vi "AdamsEncoderTest.vi"(10 "FW2DevRef":T1={"DevStatus"={"status"=FALSE, "code"=0, "source"=""}, "EncoderIndex"=enum."Invalid", "CounterIndex"=enum."Ctr 1", "DistancePerCount"=2.0, "Decoding Type"=enum."4x"}, 11 "FW1DevRef":T1={"DevStatus"={"status"=FALSE, "code"=0, "source"=""}, "EncoderIndex"=enum."Invalid", "CounterIndex"=enum."Ctr 1", "DistancePerCount"=2.0, "Decoding Type"=enum."4x"}) -> (2 "FW2Change":dbl, 3 "FW1Change":dbl)   [LabVIEW 2014]
uses:
  <vilib>/Rock Robotics/WPI/Encoder/WPI_EncoderDevRef.ctl
  <vilib>/Rock Robotics/SystemInterfaces/Encoder/FPGA_EncoderIdx.ctl
  <vilib>/Rock Robotics/SystemInterfaces/Counter/FPGA_CounterCtrSystemIndex.ctl
  <vilib>/Rock Robotics/WPI/Encoder/WPI_EncoderType.ctl
panel:
  in  "Change each time":dbl
  in  "FW2Rate":dbl
  in  "FW1Rate":dbl
  in  "DiffConstant":dbl
  in  "OffSetState":T5(ring)
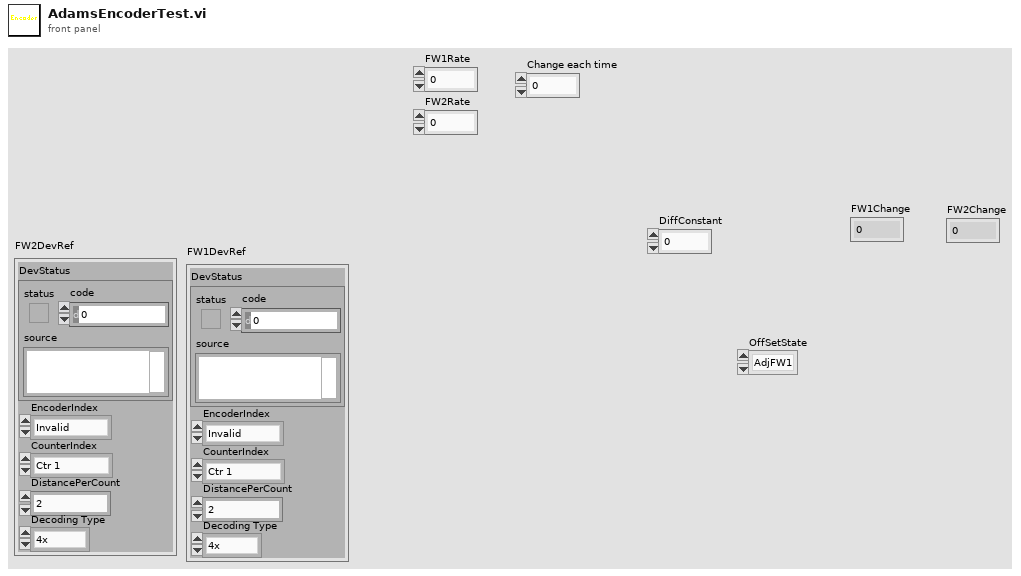
[diagram p1: front panel]
types:
  T1 = typedef "WPI_EncoderDevRef.ctl" = cluster{"DevStatus":errorcluster, "EncoderIndex":T2, "CounterIndex":T3, "DistancePerCount":dbl, "Decoding Type":T4}
  T2 = typedef "FPGA_EncoderIdx.ctl" = enum8{"Enc 0", "Enc 1", "Enc 2", "Enc 3", "Enc 4", "Enc 5", "Enc 6", "Enc 7", "Invalid"}
  T3 = typedef "FPGA_CounterCtrSystemIndex.ctl" = enum8{"Ctr 0", "Ctr 1", "Ctr 2", "Ctr 3", "Ctr 4", "Ctr 5", "Ctr 6", "Ctr 7", "Invalid"}
  T4 = typedef "WPI_EncoderType.ctl" = enum16{"1x", "2x", "4x"}
  T5 = enum16{"AdjFW1", "AdjFW2", "FW2H", "FW1H", "Equal"}
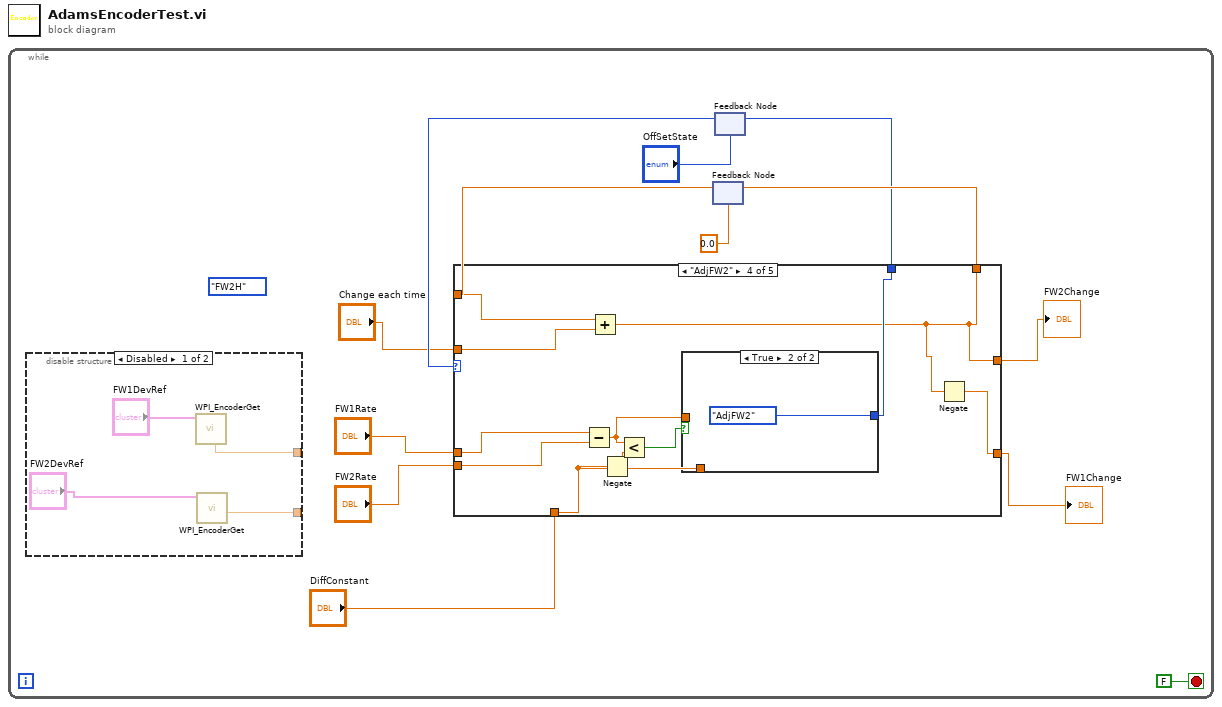
[diagram p0: block diagram]
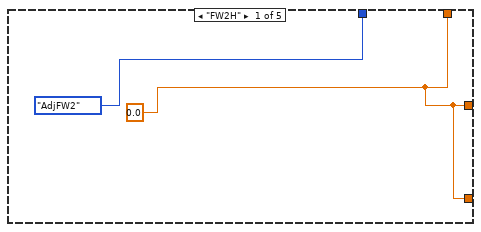
[diagram p3: hidden frame]
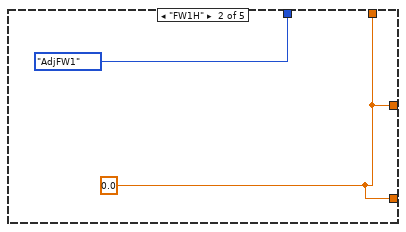
[diagram p4: hidden frame]
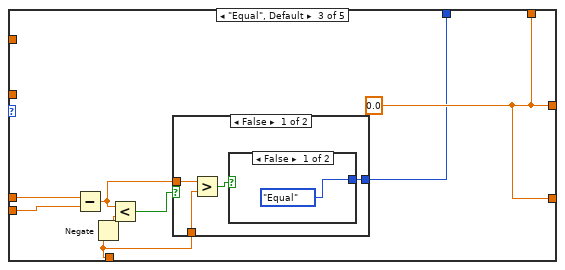
[diagram p5: hidden frame]
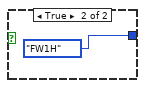
[diagram p6: hidden frame]
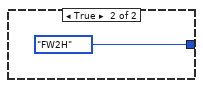
[diagram p7: hidden frame]
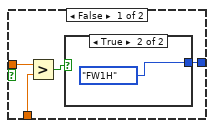
[diagram p8: hidden frame]
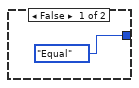
[diagram p9: hidden frame]
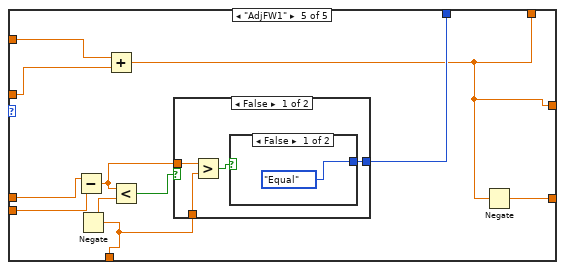
[diagram p10: hidden frame]
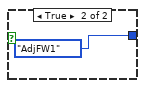
[diagram p11: hidden frame]
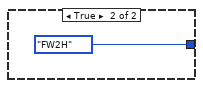
[diagram p12: hidden frame]
diagram:
  n1 = while {
    stop <- FALSE stop-if-true
    (unwired) T5."FW2H" ("OffSetState")
    n2 = disable-structure shown="Disabled" {
      disable-tunnel: [w15 _] -> _
      disable-tunnel: [w14 _] -> _
      frame Disabled {
        n3 = call <vilib>:"WPI_EncoderGet.vi"("EncoderDevRef"="FW1DevRef") -> ("Rate"=w15:dbl)  [unwired: 5 in, 5 out]
        n4 = call <vilib>:"WPI_EncoderGet.vi"("EncoderDevRef"="FW2DevRef") -> ("Rate"=w14:dbl)  [unwired: 5 in, 5 out]
      }
      frame Enabled {
      }
    }
    n5 = feedback #1(0.0) -> (w10:dbl)
    n6 = feedback #2("OffSetState") -> (w7:T5)
    n7 = case shown="\"AdjFW2\"" w7 {
      tunnel: [w19 w21 w29 w38 w57] -> w13
      tunnel: [w19 w21 w29 w40 w56] -> w12
      tunnel: w10 -> [_ _ _ w39 w58]
      tunnel: [w19 w21 w29 w38 w57] -> w9
      tunnel: "FW1Rate" -> [_ _ w28 w44 w62]
      tunnel: "FW2Rate" -> [_ _ w27 w43 w61]
      tunnel: "DiffConstant" -> [_ _ w23 w42 w60]
      tunnel: [T5."AdjFW2" ("OffSetState") T5."AdjFW1" ("OffSetState") w22 w41 w59] -> w5
      tunnel: "Change each time" -> [_ _ _ w37 w55]
      frame "FW2H" {
        w19 = 0.0
      }
      frame "FW1H" {
        w21 = 0.0
      }
      frame "Equal", Default {
        w29 = 0.0
        n8 = Subtract(x=w28, y=w27) -> (x-y=w25:dbl)
        n9 = Negate(x=w23) -> (-x=w24:dbl)
        n10 = Less?(x=w25, y=w24) -> (x < y?=w26:bool)
        n11 = case shown="False" w26 {
          tunnel: w25 -> [w32 _]
          tunnel: w23 -> [w31 _]
          tunnel: [w30 T5."FW2H" ("OffSetState")] -> w22
          frame False {
            n12 = Greater?(x=w32, y=w31) -> (0:w33:bool)
            n13 = case shown="False" w33 {
              tunnel: [T5."Equal" ("OffSetState") T5."FW1H" ("OffSetState")] -> w30
              frame False {
              }
              frame True {
              }
            }
          }
          frame True {
          }
        }
      }
      frame "AdjFW2" {
        n14 = Subtract(x=w44, y=w43) -> (x-y=w46:dbl)
        n15 = Add(x=w39, y=w37) -> (x+y=w38:dbl)
        n16 = Negate(x=w42) -> (-x=w45:dbl)
        n17 = Less?(x=w46, y=w45) -> (x < y?=w47:bool)
        n18 = case shown="True" w47 {
          tunnel: w46 -> [w50 _]
          tunnel: w42 -> [w49 _]
          tunnel: [w48 T5."AdjFW2" ("OffSetState")] -> w41
          frame False {
            n19 = Greater?(x=w50, y=w49) -> (0:w51:bool)
            n20 = case shown="True" w51 {
              tunnel: [T5."Equal" ("OffSetState") T5."FW1H" ("OffSetState")] -> w48
              frame False {
              }
              frame True {
              }
            }
          }
          frame True {
          }
        }
        n21 = Negate(x=w38) -> (-x=w40:dbl)
      }
      frame "AdjFW1" {
        n22 = Subtract(x=w62, y=w61) -> (x-y=w64:dbl)
        n23 = Negate(x=w60) -> (-x=w63:dbl)
        n24 = Add(x=w58, y=w55) -> (x+y=w57:dbl)
        n25 = Less?(x=w64, y=w63) -> (x < y?=w65:bool)
        n26 = case shown="False" w65 {
          tunnel: w64 -> [w68 _]
          tunnel: w60 -> [w67 _]
          tunnel: [w66 T5."FW2H" ("OffSetState")] -> w59
          frame False {
            n27 = Greater?(x=w68, y=w67) -> (0:w69:bool)
            n28 = case shown="False" w69 {
              tunnel: [T5."Equal" ("OffSetState") T5."AdjFW1" ("OffSetState")] -> w66
              frame False {
              }
              frame True {
              }
            }
          }
          frame True {
          }
        }
        n29 = Negate(x=w57) -> (-x=w56:dbl)
      }
    }
    "FW1Change" <- w12
    "FW2Change" <- w13
    n30 = feedback-in #1(w9) -> ()
    n31 = feedback-in #2(w5) -> ()
  }
